vi "Practica 2.vi"() -> ()   [LabVIEW 2020]
uses:
  <vilib>/express/express shared/transition.llb/Dynamic To Waveform Array.vi
  <vilib>/express/express signal manip/GetorSetDDTAttributes/Set DDT Attributes/SetT0.vi
  <vilib>/express/express shared/transition.llb/Waveform Array To Dynamic.vi
  <vilib>/express/express signal manip/GetorSetDDTAttributes/Set DDT Attributes/Set DDT Properties.xnode
panel:
  in  "Escribir archivo":bool=TRUE caption="Flush? (T)"
  out "Min & Max":bool
  out "Señal filtrada":dbl[](graph)
  in  "Maximo":dbl
  in  "Minimo":dbl
  out "Grafica de Min y Max":dbl[](graph)
  out "Frecuencia":dbl format="%#_13g"
  out "Señal original":dynamicdata(graph)
  in  "?":bool
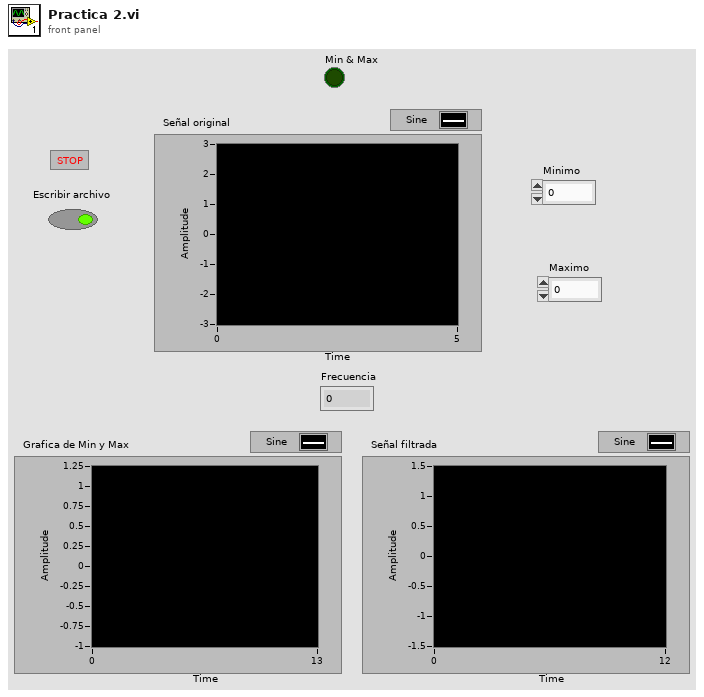
[diagram p1: front panel]
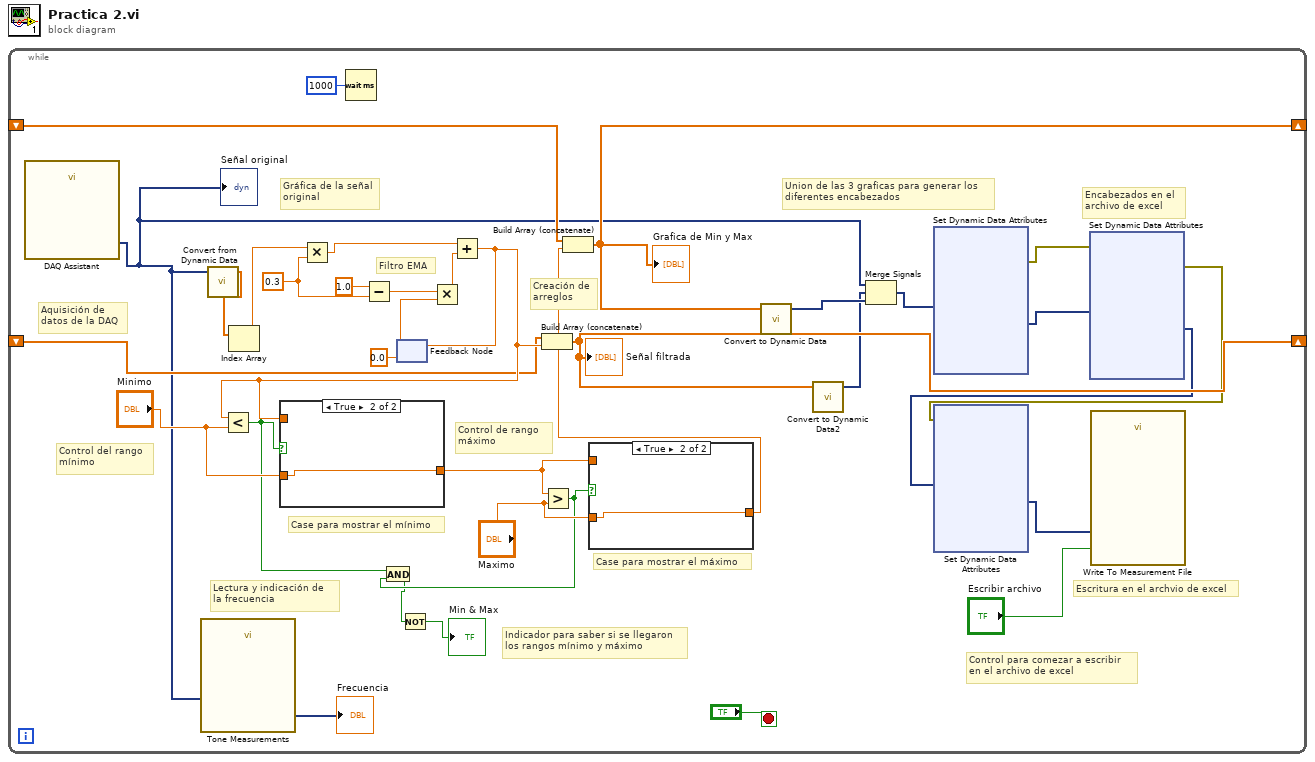
[diagram p0: block diagram]
diagram:
  n1 = while {
    shift-right: [w16] -> _
    shift-left: _ -> [w24]
    shift-right: [w14] -> _
    shift-left: _ -> [w13]
    stop <- "?" stop-if-true
    w33 = 0.3 ("y")
    # "Lectura y indicación de \nla frecuencia"
    # "Creación de\narreglos"
    # "Control para comezar a escribir \nen el archivo de excel"
    # "Escritura en el archvio de excel"
    # "Encabezados en el \narchivo de excel"
    # "Union de las 3 graficas para generar los \ndiferentes encabezados"
    # "Case para mostrar el máximo"
    # "Case para mostrar el mínimo"
    # "Indicador para saber si se llegaron \nlos rangos mínimo y máximo"
    # "Control de rango \nmáximo"
    # "Control del rango\nmínimo"
    # "Gráfica de la señal\noriginal"
    # "Filtro EMA"
    # "Aquisición de\ndatos de la DAQ"
    n2 = call "DAQ Assistant"() -> ("data"=w1:dynamicdata)  [unwired: 16 in, 3 out]
    "Señal original" <- w1
    n3 = call "Tone Measurements"("Signals"=w1) -> ("Frequency"=→"Frecuencia":dynamicdata)  [unwired: 9 in, 1 out]
    n4 = call "Convert from Dynamic Data"("Dynamic Data Type"=w1) -> ("Array"=w26:dbl[])  [unwired: 3 in]
    n5 = Index Array(array=w26) -> (element=w25:dbl)  [unwired: 1 in]
    n6 = Multiply(x=w25, y=w33) -> (x*y=w29:dbl)
    n7 = Wait (ms)(milliseconds to wait=u32 1000) -> ()  [unwired: 1 out]
    n8 = Subtract(x=1.0, y=w33) -> (x-y=w31:dbl)
    n9 = feedback #1(0.0) -> (w28:dbl)
    n10 = Multiply(x=w31, y=w28) -> (x*y=w30:dbl)
    n11 = Add(x=w29, y=w30) -> (x+y=w15:dbl)
    n12 = Less?(x=w15, y="Minimo") -> (x < y?=w18:bool)
    n13 = case shown="True" w18 {
      tunnel: "Minimo" -> [_ w81]
      tunnel: [w80 w81] -> w20
      tunnel: w15 -> [w80 _]
      frame False {
      }
      frame True {
      }
    }
    n14 = feedback-in #1(w15) -> ()
    n15 = Build Array (concatenate)(w13, w15) -> (w14:dbl[])
    "Señal filtrada" <- w14
    n16 = Greater?(x=w20, y="Maximo") -> (0:w17:bool)
    n17 = And(x=w18, y=w17) -> (x .and. y?=w12:bool)
    n18 = Not(x=w12) -> (.not. x?=→"Min & Max":bool)
    n19 = case shown="True" w17 {
      tunnel: "Maximo" -> [_ w79]
      tunnel: [w78 w79] -> w19
      tunnel: w20 -> [w78 _]
      frame False {
      }
      frame True {
      }
    }
    n20 = Build Array (concatenate)(w24, w19) -> (w16:dbl[])
    "Grafica de Min y Max" <- w16
    n21 = call "Convert to Dynamic Data"("Array"=w16) -> ("Dynamic Data Type"=w5:dynamicdata)  [unwired: 3 in]
    n22 = call "Convert to Dynamic Data2"("Array"=w14) -> ("Dynamic Data Type"=w4:dynamicdata)  [unwired: 3 in]
    n23 = Merge Signals(w1, w4, w5) -> (w6:dynamicdata)
    n24 = xnode "Set Dynamic Data Attributes"("Signals In"=w6) -> ("Signals Out"=w2:dynamicdata, "error out"=w3:errorcluster)  [unwired: 3 in]
    n25 = xnode "Set Dynamic Data Attributes"("Signals In"=w2, "error in"=w3) -> ("Signals Out"=w8:dynamicdata, "error out"=w7:errorcluster)  [unwired: 2 in]
    n26 = xnode "Set Dynamic Data Attributes"("Signals In"=w8, "error in"=w7) -> ("Signals Out"=w9:dynamicdata)  [unwired: 2 in, 1 out]
    n27 = call "Write To Measurement File"("Signals"=w9, "Flush? (T)"="Escribir archivo") -> ()  [unwired: 15 in, 3 out]
  }
